vi "WriteDigitizerConfig(SubVI).vi"(8 "error in (no error)":errorcluster, 10 "FLImDAQ":T1 {"trigger delay" format="%^#.4e"; "trigger level" min=0.0 max=3.5 step=0.5 format="%.2f"; "vertical offset" format="%.4f"; "vertical range" format="%.2f"; "min sample rate" format="%#.2p"}, 11 "appended path":path) -> (0 "error out":errorcluster)   [LabVIEW 2020]
uses:
  FLImDAQ.ctl
  <instrlib>/niScope/Controls/niScope trigger source.ctl
  <vilib>/Utility/file.llb/Write Delimited Spreadsheet (string).vi
  <vilib>/addons/_JKI.lib/Serialization/JSON/JKI JSON Serialization.lvlib
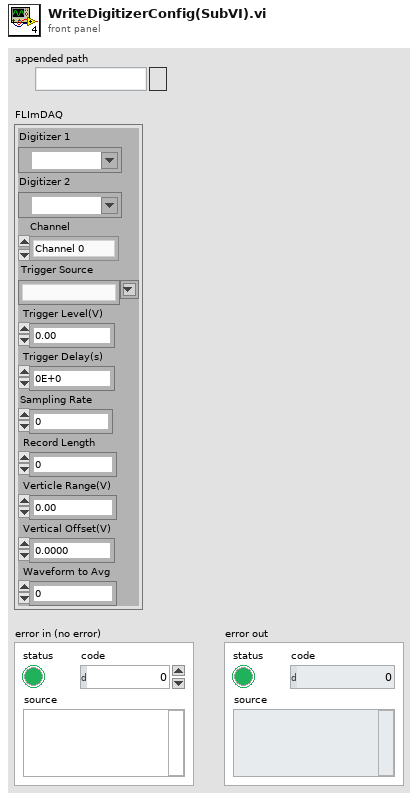
[diagram p1: front panel]
types:
  T1 = typedef "FLImDAQ.ctl" = cluster{"Digitizer 1":refnum<k15>, "Digitizer 2":refnum<k15>, "Channel":enum16{"Channel 0", "Channel 1", "Channel 0&1"}, "trigger source":T2, "trigger level":dbl, "trigger delay":dbl, "min sample rate":dbl, "min record length":i32, "vertical range":dbl, "vertical offset":dbl, "Waveform to Avg":i16}
  T2 = typedef "niScope trigger source.ctl" = string
  T3 = cluster{"Digitizer1":string, "Digitizer2":string, "Channel":enum16{"Channel 0", "Channel 1", "Channel 0&1"}, "trigger source":T2, "trigger level":dbl, "trigger delay":dbl, "min sample rate":dbl, "min record length":i32, "vertical range":dbl, "vertical offset":dbl, "Waveform to Avg":i32}
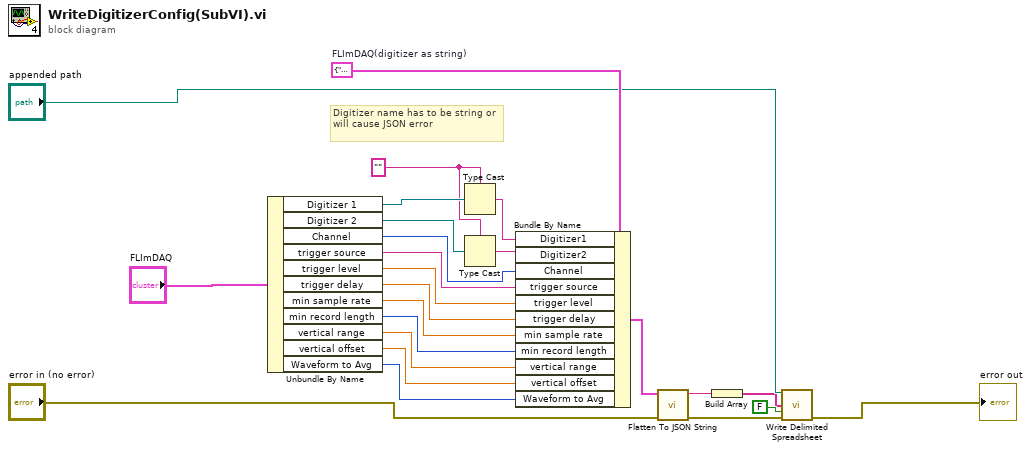
[diagram p0: block diagram]
diagram:
  w11 = T3 {"Digitizer1"="", "Digitizer2"="", "Channel"=enum."Channel 0", "trigger source"="VAL_EXTERNAL", "trigger level"=0.5, "trigger delay"=1.35e-07, "min sample rate"=12500000000.0, "min record length"=2500, "vertical range"=1.0, "vertical offset"=-0.25, "Waveform to Avg"=2000}  # FLImDAQ(digitizer as string)
  w10 = ""
  # "Digitizer name has to be string or will cause JSON error"
  n1 = Unbundle By Name("FLImDAQ") -> ("Digitizer 1"=w14:refnum<k15>, "Digitizer 2"=w9:refnum<k15>, "Channel"=w15:enum16{"Channel 0", "Channel 1", "Channel 0&1"}, "trigger source"=w16:T2, "trigger level"=w17:dbl, "trigger delay"=w18:dbl, "min sample rate"=w19:dbl, "min record length"=w20:i32, "vertical range"=w21:dbl, "vertical offset"=w22:dbl, "Waveform to Avg"=w23:i16)
  n2 = Type Cast(type=w10, x=w14) -> (*(type *) &x=w12:string)
  n3 = Type Cast(type=w10, x=w9) -> (*(type *) &x=w13:string)
  n4 = Bundle By Name(cluster=w11, "Digitizer1"=w12, "Digitizer2"=w13, "Channel"=w15, "trigger source"=w16, "trigger level"=w17, "trigger delay"=w18, "min sample rate"=w19, "min record length"=w20, "vertical range"=w21, "vertical offset"=w22, "Waveform to Avg"=w23) -> (w24:T3)
  n5 = call <vilib>:"Flatten To JSON String.vi"("error in"="error in (no error)", "Variant"=w24) -> ("error out"=w6:errorcluster, "JSON String"=w3:string)  [unwired: 8 in]
  n6 = Build Array(w3) -> (w1:string[])
  n7 = call-poly <vilib>:"Write Delimited Spreadsheet.vi"("file path (dialog if empty)"="appended path", "1D data"=w1, "append to file? (new file:F)"=FALSE, "error in (no error)"=w6) -> ("error out"=→"error out":errorcluster)  [unwired: 10 in, 1 out]
